vi "Register Custom gRPC Message.vi"(8 "error in":errorcluster, 10 "gRPC ID":T1, 11 "Node in":refnum<class "AMS Cycler Template.lvclass">) -> (0 "error out":errorcluster, 3 "Node out":refnum<class "AMS Cycler Template.lvclass">)   [LabVIEW 2023, in "AMS Cycler Template.lvlib" / "AMS Cycler Template.lvclass"]
uses:
  AMS Cycler Template.lvclass
  C:/Program Files/National Instruments/LabVIEW 2024/vi.lib/ADAS Replay HIL/Template Node/Plugin/Template Node/Template Node.lvclass
  <vilib>/gRPC/LabVIEW gRPC Library/Shared/grpcId.ctl
  Custom gRPC/AMSCyclerTemplateService_server/RPC Service/AMSCyclerTemplateService/AMSCyclerTemplateService.lvclass
  C:/Program Files/National Instruments/LabVIEW 2024/vi.lib/gRPC/LabVIEW gRPC Servicer/ServiceBase/ServiceBase.lvclass
  Custom gRPC/AMSCyclerTemplateService_server/AMSCyclerTemplateService_server.lvlib
  <vilib>/ADAS Replay HIL/Template Node/Plugin/Template Node/Template Node.lvclass
  <vilib>/gRPC/LabVIEW gRPC Library/grpc-lvsupport-release.lvlib
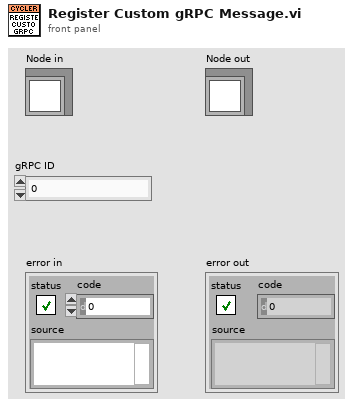
[diagram p1: front panel]
types:
  T1 = typedef "grpc-lvsupport-release.lvlib/grpcId.ctl" = u64
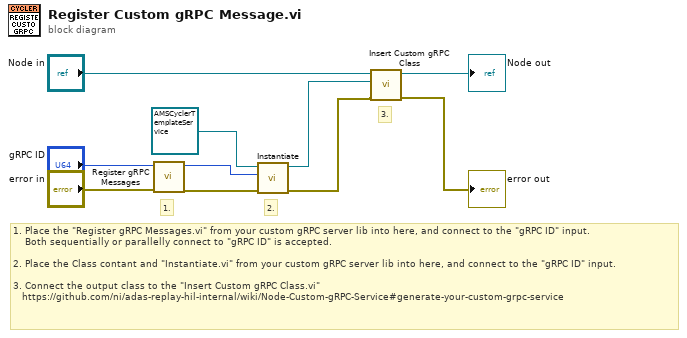
[diagram p0: block diagram]
diagram:
  # "3."
  # "2."
  # "1."
  # "1. Place the \"Register gRPC Messages.vi\" from your custom gRPC server lib into here, and connect to the \"gRPC ID\" input.\n    Both sequentially or parallelly connect to \"gRPC ID\" is accepted.\n\n2. Place the Class contant and \"Instantiate.vi\" from your custom gRPC server lib into here, and connect to the \"gRPC ID\" input.\n\n3. Connect the output class to the \"Insert Custom gRPC Class.vi\"\n   https://github.com/ni/adas-replay-hil-internal/wiki/Node-Custom-gRPC-Service#generate-your-custom-grpc-service"
  n1 = call "Register gRPC Messages.vi"("error in (no error)"="error in", "gRPC ID"="gRPC ID") -> ("error out"=w7:errorcluster, "gRPC ID Out"=w6:T1)  [unwired: 8 in]
  n2 = call-dynamic "Instantiate.vi"("error in"=w7, "gRPCid"=w6, "iService"=refnum<class "AMSCyclerTemplateService.lvclass"> refnum ("gRPC-servicer.lvlib:iService.lvclass")) -> ("error out"=w3:errorcluster, "iService"=w4:refnum<class "AMSCyclerTemplateService.lvclass">)  [unwired: 7 in]
  n3 = call <vilib>:"Insert Custom gRPC Class.vi"("error in"=w3, "Custom gRPC Class"=w4, "Node in"="Node in") -> ("error out"=→"error out":errorcluster, "Node out"=→"Node out":refnum<class "AMS Cycler Template.lvclass">)  [unwired: 7 in]
